vi "Init with new document.vi"(0 "Device In":T1, 5 "Name In":string, 11 "error in":errorcluster) -> (4 "Device Out":T1, 6 "id":string, 15 "error out":errorcluster)   [LabVIEW 2019]
uses:
  <userlib>/IoT Devices/_subVIs/HTTPComm.ctl
  _SubVI/Cluster.ctl
panel:
  out "Comm":T2
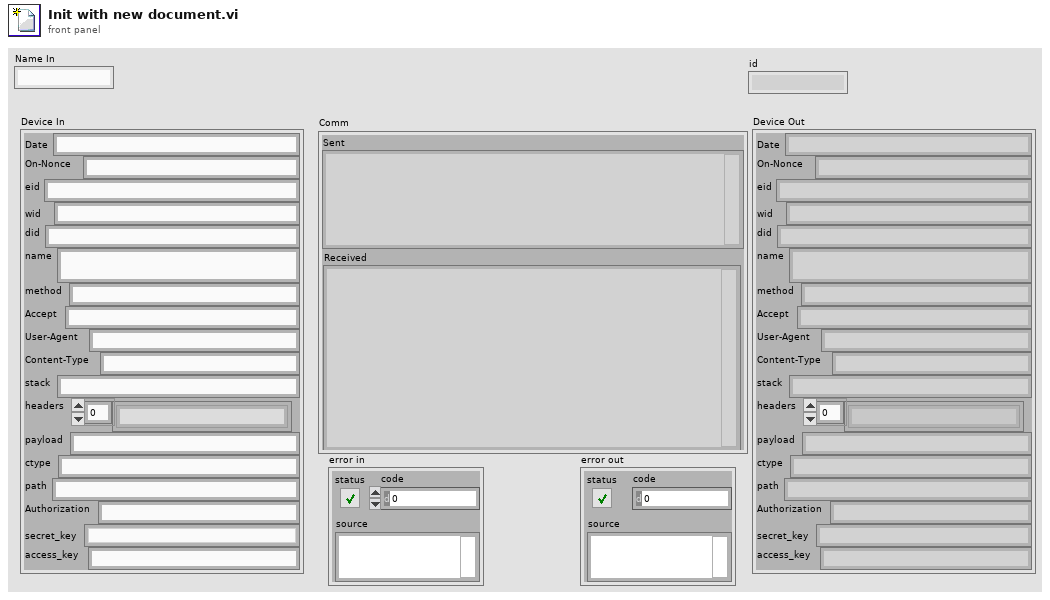
[diagram p1: front panel]
types:
  T1 = typedef "Cluster.ctl" = cluster{"Date":string, "On-Nonce":string, "eid":string, "wid":string, "did":string, "name":string, "method":string, "Accept":string, "User-Agent":string, "Content-Type":string, "stack":string, "headers":string[], "payload":string, "ctype":string, "path":string, "Authorization":string, "secret_key":string, "access_key":string}
  T2 = typedef "HTTPComm.ctl" = cluster{"url":string, "sent headers":string, "sent body":string, "headers":string, "body":string, "Sent":string, "Received":string}
  T3 = cluster{"name":string, "defaultWorkspace":cluster{"documentId":string, "id":string}}
  T4 = cluster{"name":string, "ownerType":i32, "isPublic":bool}
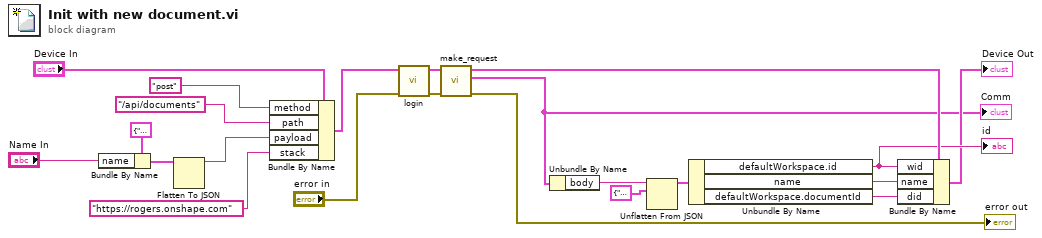
[diagram p0: block diagram]
diagram:
  n1 = Bundle By Name(cluster=T4 {"name"="", "ownerType"=0, "isPublic"=FALSE}, "name"="Name In") -> (w21:T4)
  n2 = Flatten To JSON(anything=w21) -> (JSON string=w17:string)  [unwired: 2 in, 1 out]
  n3 = Bundle By Name(cluster="Device In", "method"="post" ("Method"), "path"="/api/documents" ("payload"), "payload"=w17, "stack"="https://rogers.onshape.com" ("stacks")) -> (w11:T1)
  n4 = call "login.vi"("error in"="error in", "Device In"=w11) -> ("error out"=w9:errorcluster, "Device Out"=w10:T1)  [unwired: 8 in]
  n5 = call "make_request.vi"("Error in"=w9, "Device In"=w10) -> ("error out"=→"error out":errorcluster, "Comm"=w2:T2, "Device Out"=w12:T1)  [unwired: 7 in]
  "Comm" <- w2
  n6 = Unbundle By Name(w2) -> ("body"=w14:string)
  n7 = Unflatten From JSON(JSON string=w14, type and defaults=T3 {"name"="", "defaultWorkspace"={"documentId"="", "id"=""}}) -> (value=w13:T3)  [unwired: 5 in, 1 out]
  n8 = Unbundle By Name(w13) -> ("defaultWorkspace.id"=w6:string, "name"=w8:string, "defaultWorkspace.documentId"=w7:string)
  "id" <- w6
  n9 = Bundle By Name(cluster=w12, "wid"=w6, "name"=w8, "did"=w7) -> (→"Device Out":T1)
